vi "Match time constant to value.vi"(1 "Time constant":dbl[unit]) -> (0 "Tau":T1 items=["10 us", "30 us", "100 us", "300 us", "1 ms", "3 ms", "10 ms", "30 ms", "100 ms", "300 ms", "1 s", "3 s", "10 s", "30 s", "100 s", "300 s", "1 ks", "3 ks", "10 ks", "30 ks"])   [LabVIEW 2017, in "SR830.lvlib"]
uses:
  Tau.ctl
  SR830.lvlib
panel:
  # "Time constant must be multiples of 10 or 3..."
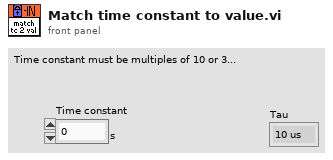
[diagram p1: front panel]
types:
  T1 = typedef "SR830.lvlib/Tau.ctl" = u16
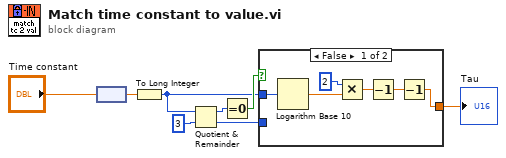
[diagram p0: block diagram]
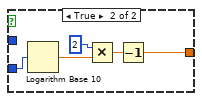
[diagram p2: hidden frame]
diagram:
  n1 = node("Time constant") -> (w7:dbl)
  n2 = To Long Integer(number=w7) -> (32bit integer=w1:i32)
  n3 = Quotient & Remainder(x=w1, y=3) -> (x-y*floor(x/y)=w5:i32, floor(x/y)=w3:i32)
  n4 = Equal To 0?(x=w5) -> (x = 0?=w4:bool)
  n5 = case shown="False" w4 {
    tunnel: w3 -> [_ w19]
    tunnel: [w9 w15] -> w2
    tunnel: w1 -> [w14 _]
    frame False {
      n6 = Logarithm Base 10(1:w14) -> (0:w11:dbl)
      n7 = Multiply(x=2, y=w11) -> (x*y=w12:dbl)
      n8 = Decrement(x=w12) -> (x-1=w10:dbl)
      n9 = Decrement(x=w10) -> (x-1=w9:dbl)
    }
    frame True {
      n10 = Logarithm Base 10(1:w19) -> (0:w18:dbl)
      n11 = Multiply(x=2, y=w18) -> (x*y=w16:dbl)
      n12 = Decrement(x=w16) -> (x-1=w15:dbl)
    }
  }
  "Tau" <- w2
